vi "Fir_reconfig.vi"(5 "new shift":i32, 6 "reset":bool, 7 "new coeffs":fxp<+/-,18,18>[](array[numeric]), 8 "valid in":bool, 9 "Q in":fxp<+/-,16,14>, 10 "I in":fxp<+/-,16,14>, 11 "new coeffs":bool) -> (0 "valid out":bool, 1 "Q out":fxp<+/-,16,14>, 2 "I out":fxp<+/-,16,14>, 4 "ready for input":bool)   [LabVIEW 2013]
uses:
  <vilib>/rvi/FXPMathLib/FxpConvert/subVIs/nifxpmath_Convert_SimConfig.ctl
  <vilib>/fxp/LVFixedPointQuantizationPolicyTypeDef.ctl
  <vilib>/fxp/LVFixedPointOverflowPolicyTypeDef.ctl
  <vilib>/rvi/IPIntegrationNode/IPINode_Utilities/niFpgaIPINodeSimCore.vi
  <vilib>/rvi/FXPMathLib/FxpConvert/simVIs/DllFxpConvertTemp_sub.vi
  <vilib>/rvi/XilinxIP/XIPIN_XNode/niFpgaXIPIN.xnode
  C:/Users/Public/Documents/LabVIEW-proj/PXIe/Workspace/Filters/FIR_reconfig/FIR_reconfig_C7DB4901E5B34DF5AA9089C2303BD932.dll
  <vilib>/rvi/IPIntegrationNode/IPINode_Xnode/niFpgaIPINode.xnode
  <vilib>/rvi/FXPMathLib/FxpInterpret/XNode/nifxpmath_Interpret.xnode
  <vilib>/rvi/FXPMathLib/FxpConvert/XNode/nifxpmath_Convert.xnode
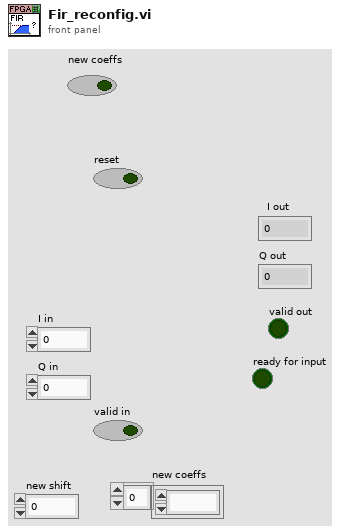
[diagram p1: front panel]
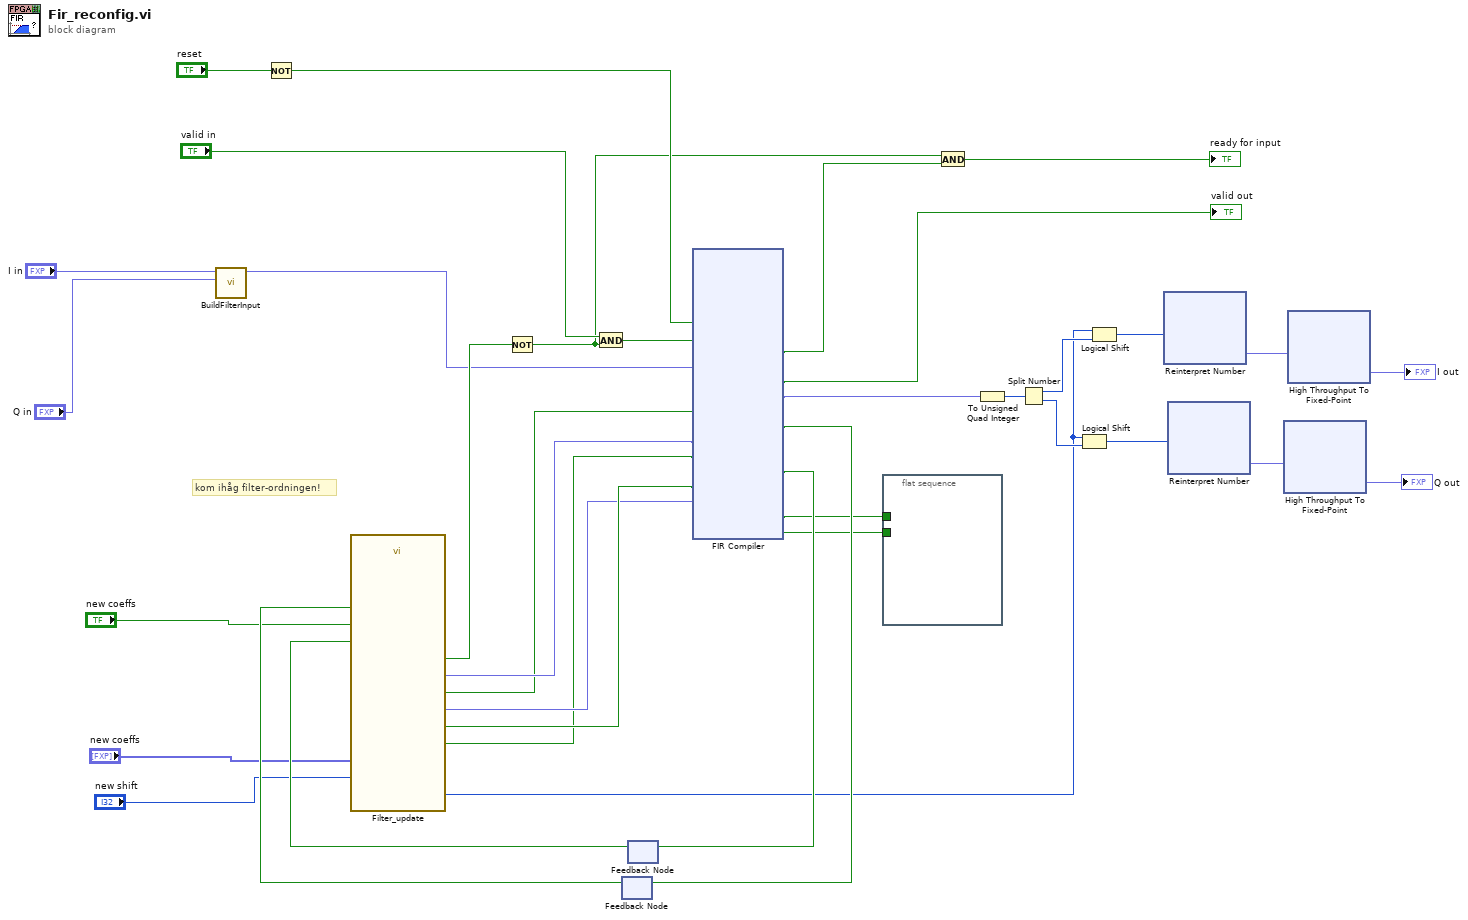
[diagram p0: block diagram]
diagram:
  # "kom ihåg filter-ordningen!"
  n1 = call "BuildFilterInput.vi"("Q in"="Q in", "I in"="I in") -> ("Filter input"=w18:fxp<+,32,32>)  [unwired: 9 in]
  n2 = Not(x="reset") -> (.not. x?=w30:bool)
  n3 = feedback #1() -> (w35:bool)  [unwired: 1 in]
  n4 = feedback #2() -> (w36:bool)  [unwired: 1 in]
  n5 = call "Filter_update.vi"(0:"new coeffs"="new coeffs", "new shift"="new shift", 2:"new coeffs"="new coeffs", "config rdy for data"=w35, "reload rdy for data"=w36) -> ("busy"=w32:bool, "s_axis_reload_tlast"=w25:bool, "s_axis_config_tvalid"=w21:bool, "shift out"=w1:i32, "s_axis_config_tdata"=w22:fxp<+,8,8>, "s_axis_reload_tvalid"=w23:bool, "s_axis_reload_tdata"=w24:fxp<+,24,24>)  [unwired: 8 in]
  n6 = Not(x=w32) -> (.not. x?=w15:bool)
  n7 = And(x="valid in", y=w15) -> (x .and. y?=w29:bool)
  n8 = xnode ("FIR Compiler")("aresetn"=w30, "s_axis_data_tvalid"=w29, "s_axis_data_tdata"=w18, "s_axis_config_tvalid"=w21, "s_axis_config_tdata"=w22, "s_axis_reload_tvalid"=w23, "s_axis_reload_tlast"=w25, "s_axis_reload_tdata"=w24) -> ("s_axis_data_tready"=w14:bool, "m_axis_data_tvalid"=→"valid out":bool, "m_axis_data_tdata"=w9:fxp<+,64,64>, "s_axis_config_tready"=w27:bool, "s_axis_reload_tready"=w26:bool, "event_s_reload_tlast_missing"=w17:bool, "event_s_reload_tlast_unexpected"=w16:bool)  [unwired: 1 in]
  n9 = feedback-in #1(w27) -> ()
  n10 = feedback-in #2(w26) -> ()
  n11 = flat-sequence {
    tunnel: w17 -> [_]
    tunnel: w16 -> [_]
    frame #0 {
    }
  }
  n12 = And(x=w15, y=w14) -> (x .and. y?=→"ready for input":bool)
  n13 = To Unsigned Quad Integer(1:w9) -> (0:w12:u64)
  n14 = Split Number(x=w12) -> (hi(x)=w4:u32, lo(x)=w6:u32)
  n15 = Logical Shift(y=w1, x=w6) -> (x << y=w5:u32)
  n16 = Logical Shift(y=w1, x=w4) -> (x << y=w3:u32)
  n17 = xnode "Reinterpret Number"("x"=w3) -> ("y"=w10:fxp<+/-,32,23>)
  n18 = xnode "Reinterpret Number"("x"=w5) -> ("y"=w11:fxp<+/-,32,23>)
  n19 = xnode "High Throughput To Fixed-Point"("x"=w11) -> ("y"=→"Q out":fxp<+/-,16,14>)
  n20 = xnode "High Throughput To Fixed-Point"("x"=w10) -> ("y"=→"I out":fxp<+/-,16,14>)
